vi "GOMDBTS2048 get TM3015 Rf by Hue.vi"(8 "error in (no error)":errorcluster, 11 "handle":i32) -> (0 "error out":errorcluster, 2 "function return":i32, 3 "RfByHue":dbl[](array[numeric]))   [LabVIEW 2015, in "GOMDBTS2048.lvlib"]
doc: "GOBTS2048DLL int __stdcall GOMDBTS2048_getTM3015Coordinates(int handle, double* TLCoordinates, double* RLCoordinates);"
uses:
  GOMDBTS2048.lvlib
  runtime/GOMDBTS2048.dll
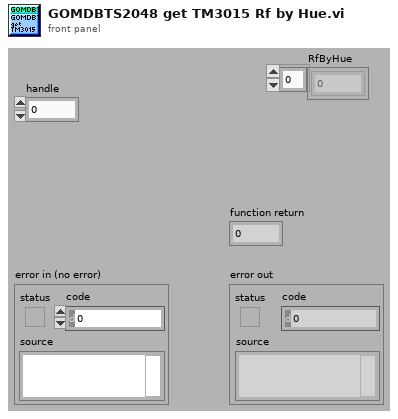
[diagram p1: front panel]
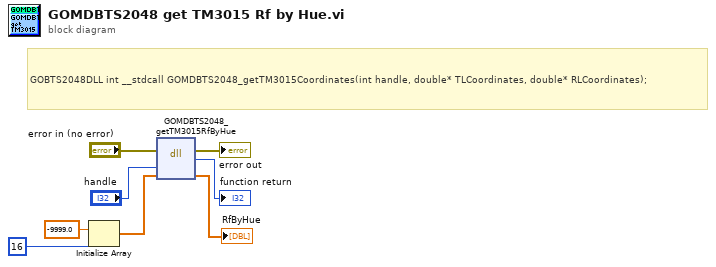
[diagram p0: block diagram]
diagram:
  # "GOBTS2048DLL int __stdcall GOMDBTS2048_getTM3015Coordinates(int handle, double* TLCoordinates, double* RLCoordinates);"
  n1 = Initialize Array(-9999.0 ("element"), 16 ("dimension size")) -> (w2:dbl[])
  n2 = dll-call lib="C:/Users/rkoch/Documents/GO_Library/runtime/GOMDBTS2048.*" fn="GOMDBTS2048_getTM3015RfByHue"(error in="error in (no error)", "handle"="handle", "RfByHue"=w2) -> (error out=→"error out":errorcluster, "return type"=→"function return":i32, "RfByHue"=→"RfByHue":dbl[])  [unwired: 3 in, 1 out]
